vi "fkcommand.vi"(0 "object in":refnum<class "212format_work.lvclass">, 1 "in":T1, 5 "error in (no error)":errorcluster) -> (14 "object out":refnum<class "212format_work.lvclass">, 15 "out":T2, 19 "error out":errorcluster)   [LabVIEW 2016, in "212format_work.lvclass"]
uses:
  212format_work.lvclass
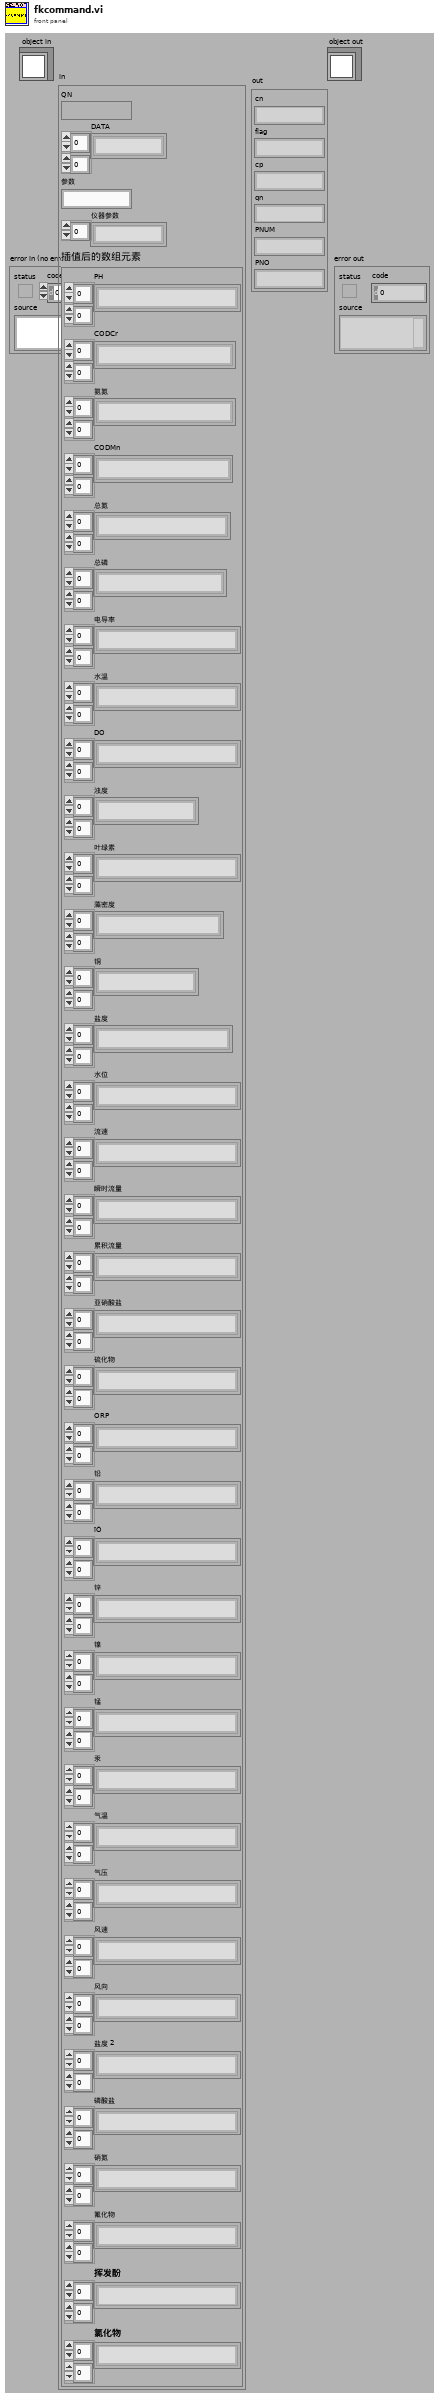
[diagram p1: front panel]
types:
  T1 = cluster{"QN":string, "DATA":string[][], "参数":string, "仪器参数":string[], "插值后的数组元素":cluster{"PH":string[][], "CODCr":string[][], "氨氮":string[][], "CODMn":string[][], "总氮":string[][], "总磷":string[][], "电导率":string[][], "水温":string[][], "DO":string[][], "浊度":string[][], "叶绿素":string[][], "藻密度":string[][], "铜":string[][], "盐度":string[][], "水位":string[][], "流速":string[][], "瞬时流量":string[][], "累积流量":string[][], "亚硝酸盐":string[][], "硫化物":string[][], "ORP":string[][], "铅":string[][], "ïÓ":string[][], "锌":string[][], "镍":string[][], "锰":string[][], "汞":string[][], "气温":string[][], "气压":string[][], "风速":string[][], "风向":string[][], "盐度 2":string[][], "磷酸盐":string[][], "硝氮":string[][], "氟化物":string[][], "挥发酚":string[][], "氯化物":string[][]}}
  T2 = cluster{"cn":string, "flag":string, "cp":string, "qn":string, "PNUM":string, "PNO":string}
  T3 = typedef "212format_work.lvclass/fkcommand控件.ctl" = cluster{"反控命令枚举":enum16{"返回请求应答", "返回执行结果"}, "执行结果定义":u16, "执行反馈":bool, "执行结果":u16, "是否判断反馈？":bool}
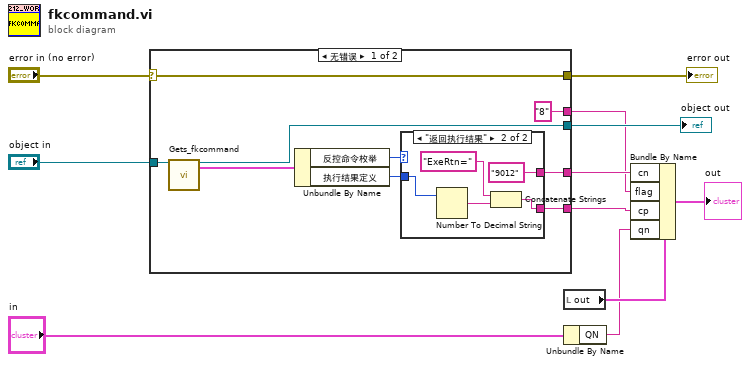
[diagram p0: block diagram]
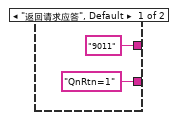
[diagram p2: hidden frame]
diagram:
  n1 = case shown="无错误" "error in (no error)" {
    selector: "error in (no error)" -> [w20 w29]
    tunnel: [w20 w29] -> w10
    tunnel: [w12 w28] -> w8
    tunnel: "object in" -> [w14 w28]
    tunnel: [w17 _] -> w3
    tunnel: [w16 _] -> w5
    tunnel: ["8" ("ST") _] -> w4
    frame No Error {
      n2 = call-dynamic "Gets_fkcommand.vi"("object in"=w14) -> ("object out"=w12:refnum<class "212format_work.lvclass">, "fkcommand"=w13:T3)  [unwired: 16 in, 1 out]
      n3 = Unbundle By Name(w13) -> ("反控命令枚举"=w19:enum16{"返回请求应答", "返回执行结果"}, "执行结果定义"=w18:u16)
      n4 = case shown="\"返回执行结果\"" w19 {
        tunnel: ["QnRtn=1" w24] -> w17
        tunnel: w18 -> [_ w25]
        tunnel: ["9011" ("CN") "9012" ("CN")] -> w16
        frame "返回请求应答", Default {
        }
        frame "返回执行结果" {
          n5 = Number To Decimal String(number=w25) -> (decimal integer string=w26:string)  [unwired: 1 in]
          n6 = Concatenate Strings("ExeRtn=", w26) -> (w24:string)
        }
      }
    }
    frame Error {
    }
  }
  "error out" <- w10
  "object out" <- w8
  n7 = local read "out"() -> (w7:T2)
  n8 = Unbundle By Name("in") -> ("QN"=w1:string)
  n9 = Bundle By Name(cluster=w7, "cn"=w5, "flag"=w4, "cp"=w3, "qn"=w1) -> (→"out":T2)
